vi "配置保存读取.vi"(8 "error in (no error)":errorcluster caption="错误输入（无错误）", 11 "配置":enum16{"读取", "写入"}(ring)) -> (0 "error out":errorcluster caption="错误输出")   [LabVIEW 2016, in "数据查询.lvlib"]
uses:
  <vilib>/Utility/config.llb/NI_LVConfig.lvlib
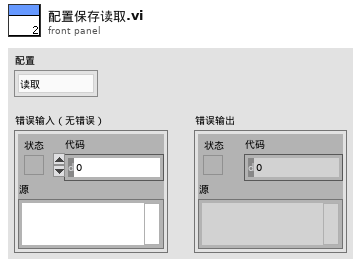
[diagram p1: front panel]
types:
  T1 = typedef "NI_LVConfig.lvlib/Config Data RefNum.ctl" = refnum<k1>
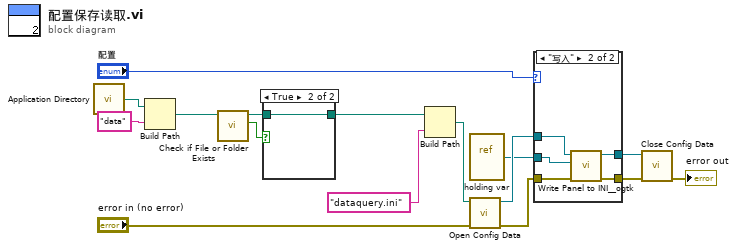
[diagram p0: block diagram]
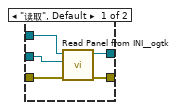
[diagram p2: hidden frame]
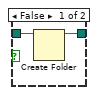
[diagram p3: hidden frame]
diagram:
  n1 = call <vilib>:"Application Directory.vi"() -> ("Application Directory"=w16:path)
  n2 = Build Path(base path=w16, name or relative path="data" ("名称或相对路径")) -> (appended path=w14:path)
  n3 = call <vilib>:"Check if File or Folder Exists.vi"("path"=w14) -> ("file or folder exists?"=w13:bool, "dup path"=w12:path)  [unwired: 8 in, 1 out]
  n4 = case shown="True" w13 {
    tunnel: w12 -> [w18 w19]
    tunnel: [w17 w19] -> w11
    frame False {
      n5 = Create Folder(path (use dialog)=w18) -> (created path=w17:path)  [unwired: 2 in, 2 out]
    }
    frame True {
    }
  }
  n6 = Build Path(base path=w11, name or relative path="dataquery.ini" ("名称或相对路径")) -> (appended path=w9:path)
  n7 = vi-ref "holding var.vi"() -> (w6:refnum<vi>)
  n8 = call <vilib>:"Open Config Data.vi"("error in (no error)"="error in (no error)", "configuration file path"=w9) -> ("error out"=w7:errorcluster, "refnum"=w8:T1)  [unwired: 7 in, 1 out]
  n9 = case shown="\"写入\"" "配置" {
    tunnel: w8 -> [w24 w29]
    tunnel: w7 -> [w23 w28]
    tunnel: w6 -> [w20 w27]
    tunnel: [w21 w26] -> w5
    tunnel: [w22 w25] -> w4
    frame "读取", Default {
      n10 = call <userlib>:"Read Panel from INI__ogtk.vi"("error in (no error)"=w23, "VI ref"=w20, "refnum"=w24) -> ("error out"=w22:errorcluster, "refnum out"=w21:T1)  [unwired: 7 in]
    }
    frame "写入" {
      n11 = call <userlib>:"Write Panel to INI__ogtk.vi"("error in (no error)"=w28, "VI ref"=w27, "refnum"=w29) -> ("error out"=w25:errorcluster, "refnum out"=w26:T1)  [unwired: 7 in]
    }
  }
  n12 = call <vilib>:"Close Config Data.vi"("error in (no error)"=w4, "refnum"=w5) -> ("error out"=→"error out":errorcluster)  [unwired: 8 in, 1 out]
